vi "sir_v4.vi"() -> ()   [LabVIEW 2009]
panel:
  in  "Sirul 2":string="LabWIEW"
  out "Numarul de caractere":dbl=17.0
  in  "stop":bool
  out "Sirul rezultat dupa concatenare":string="Aplicatie LabWIEW"
  in  "Sirul 1":string="Aplicatie "
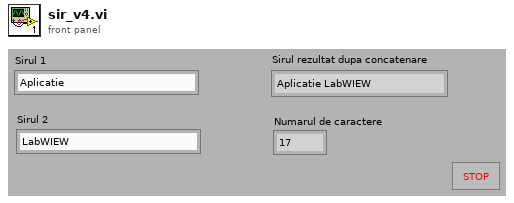
[diagram p1: front panel]
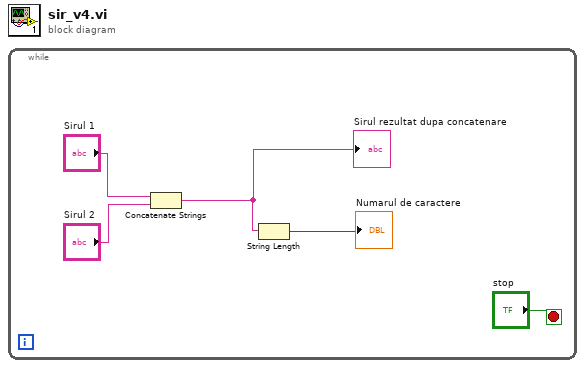
[diagram p0: block diagram]
diagram:
  n1 = while {
    stop <- "stop" stop-if-true
    n2 = Concatenate Strings("Sirul 1", "Sirul 2") -> (w1:string)
    "Sirul rezultat dupa concatenare" <- w1
    n3 = String Length(string=w1) -> (length=→"Numarul de caractere":i32)
  }
